vi "Handle Last Ack Core.vi"(4 "error in (no error)":errorcluster, 6 "Last Ack":refnum<class "Last Ack.lvclass">, 7 "Controller in":refnum<class "Controller.lvclass">) -> (0 "error out":errorcluster, 3 "Controller out":refnum<class "Controller.lvclass">)   [LabVIEW 2016, in "Controller Actor.lvlib" / "Controller.lvclass"]
doc: "(<B>Filename</B>: Actor Framework.lvlib:Actor.lvclass:Handle Last Ack Core.vi)\n\nDefines how the caller actor responds to the Last Ack message from a nested actor. The Last Ack message is the final message a nested actor sends to its caller before it shuts down. The message contains information about the final state of the nested actor.\n\nBy default, this method does nothing except return any error the nested actor sent. A descendant class may override this method to define behavior."
uses:
  Controller.lvclass
  <vilib>/ActorFramework/LastAck/Last Ack.lvclass
  <vilib>/ActorFramework/LastAck/Last Ack.lvclass/Last Ack.ctl
  Hardware/HW Config/HW Configuration.lvclass
  Hardware/Hardware.lvclass
  Hardware/HW Config/HW Configuration.lvclass/HW Configuration.ctl
  Hardware/Hardware.lvclass/Hardware.ctl
  Controller.lvclass/Controller.ctl
  <userlib>/Configuration Dialog Actor/Configuration.lvclass
  <vilib>/ActorFramework/Message Enqueuer/Message Enqueuer.lvclass/Message Enqueuer.ctl
  Measurement Actor/Measurement.lvclass
  Measurement Actor/Measurement.lvclass/Measurement.ctl
  <vilib>/ActorFramework/Message Enqueuer/Enqueue.vi
  User Interface/Messages/Enable UI Msg/Enable UI Msg.lvclass
  C:/Program Files (x86)/National Instruments/LabVIEW 2016/vi.lib/ActorFramework/Message/Message.lvclass
  <vilib>/ActorFramework/Message Priority Queue/Priority Enqueue.vi
  <vilib>/ActorFramework/Actor/Actor.lvclass
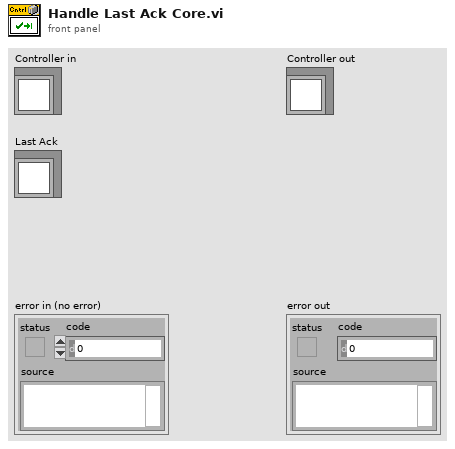
[diagram p1: front panel]
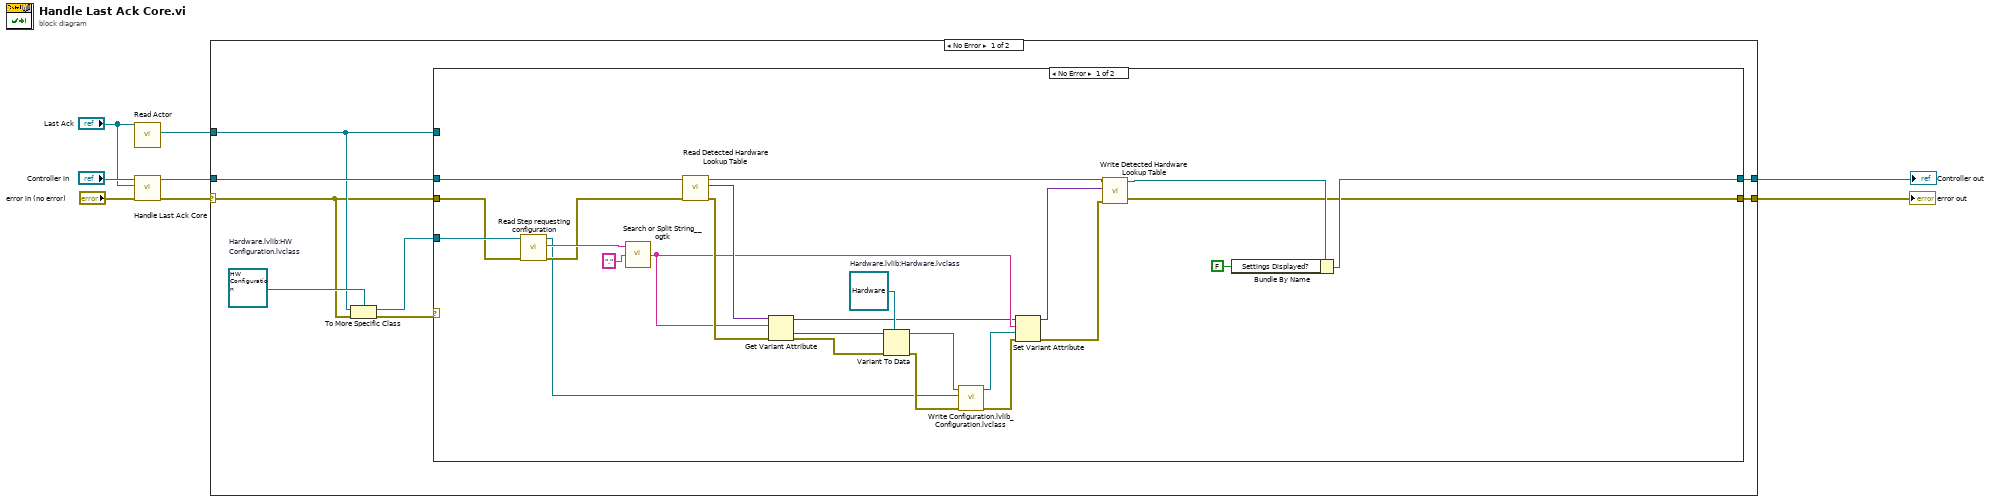
[diagram p0: block diagram]
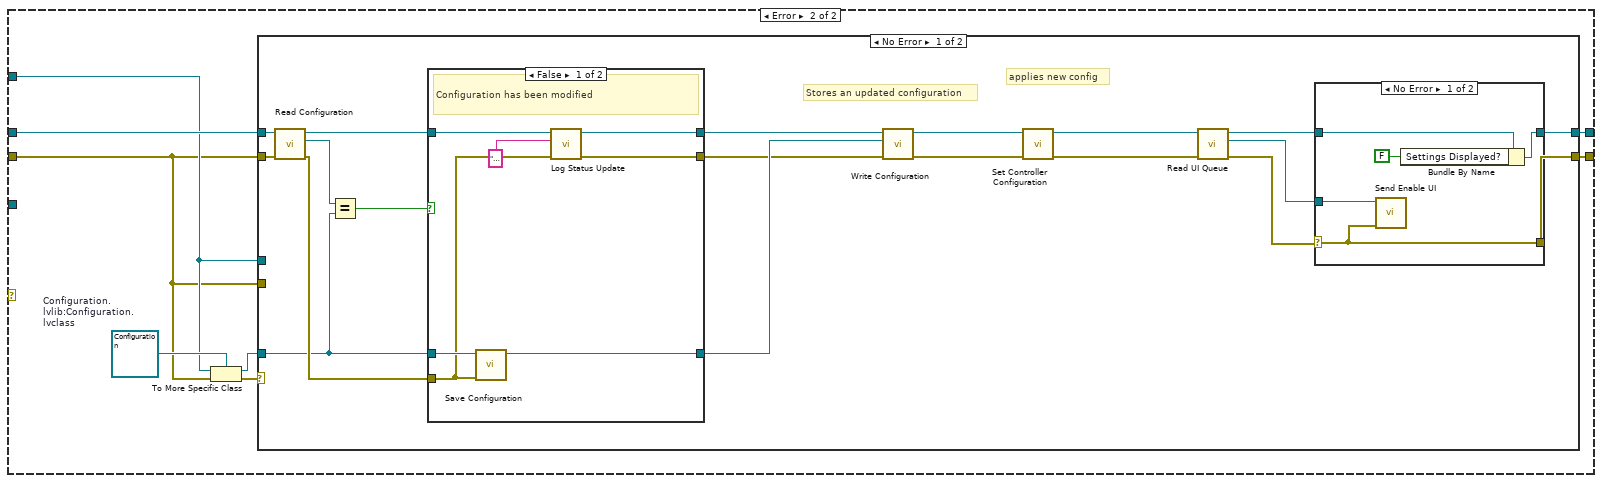
[diagram p2: hidden frame]
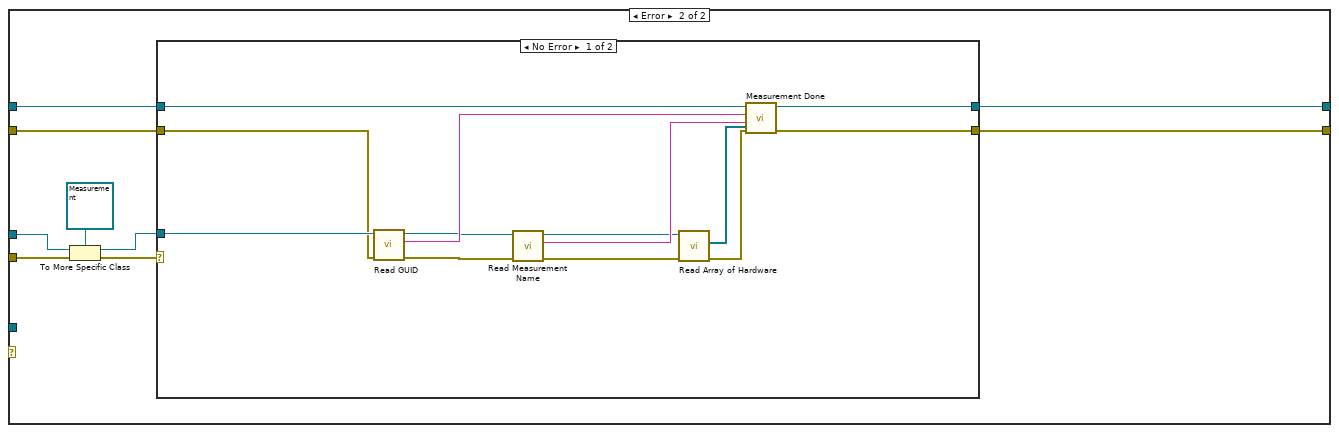
[diagram p5: hidden frame]
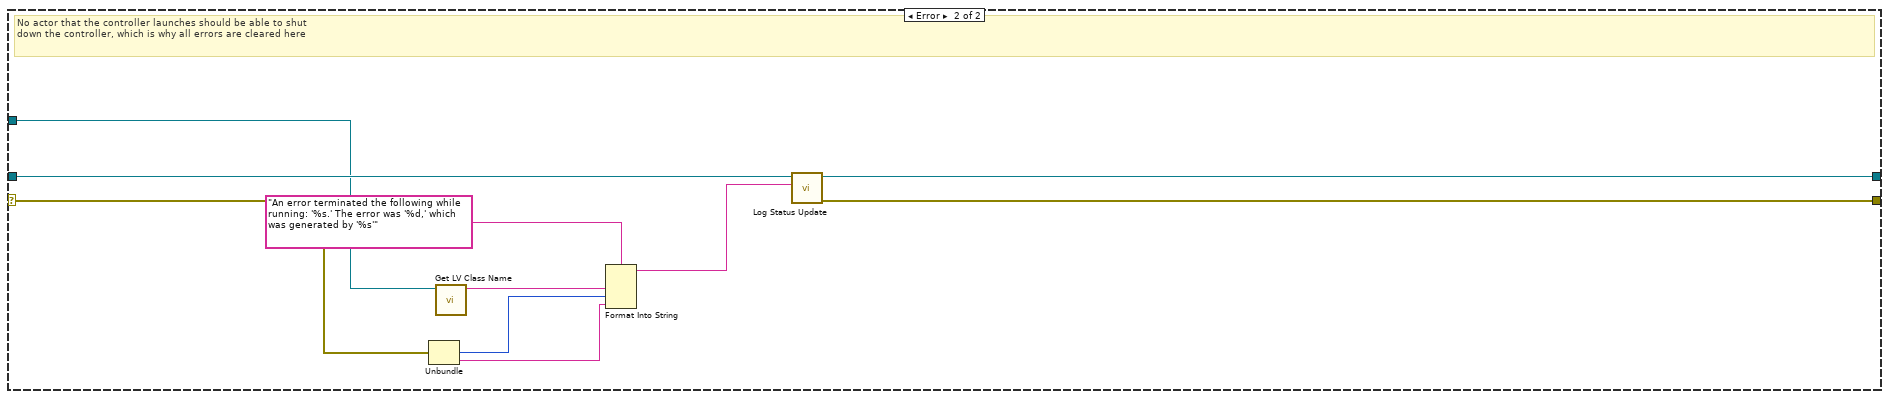
[diagram p7: hidden frame]
diagram:
  n1 = call <vilib>:"Read Actor.vi"("Last Ack"="Last Ack") -> ("Actor"=w3:refnum<class "Actor.lvclass">)  [unwired: 10 in]
  n2 = call-parent "Handle Last Ack Core.vi"("error in (no error)"="error in (no error)", "Last Ack"="Last Ack", "Actor in"="Controller in") -> ("error out"=w2:errorcluster, "Actor out"=w4:refnum<class "Controller.lvclass">)  [unwired: 3 in]
  n3 = case shown="No Error" w2 {
    selector: w2 -> [w9 w115]
    tunnel: [w16 w118] -> w7
    tunnel: [w15 w117] -> w5
    tunnel: w4 -> [w14 w119]
    tunnel: w3 -> [w12 w111]
    frame No Error {
      w13 = refnum<class "HW Configuration.lvclass"> refnum  # Hardware.lvlib:HW Configuration.lvclass
      n4 = To More Specific Class(target class=w13, reference=w12, error in=w9) -> (specific class reference=w11:refnum<class "HW Configuration.lvclass">, error out=w10:errorcluster)
      n5 = case shown="No Error" w10 {
        tunnel: [w19 w49] -> w16
        tunnel: [w18 w48] -> w15
        tunnel: w14 -> [w34 w47]
        tunnel: w12 -> [_ w43]
        tunnel: w9 -> [w40 w42]
        tunnel: w11 -> [w41 _]
        frame No Error {
          w32 = refnum<class "Hardware.lvclass"> refnum  # Hardware.lvlib:Hardware.lvclass
          n6 = call "Read Step requesting configuration.vi"("error in (no error)"=w40, "HW Configuration in"=w41) -> ("error out"=w35:errorcluster, "Step requesting configuration"=w39:string, "HW Configuration out"=w17:refnum<class "HW Configuration.lvclass">)  [unwired: 7 in]
          n7 = call <userlib>:"Search or Split String__ogtk.vi"("search string/char (-)"="." ("regular expression"), "string"=w39) -> ("substring after match"=w28:string)  [unwired: 1 in, 2 out]
          n8 = call "Read Detected Hardware Lookup Table.vi"("error in (no error)"=w35, "Controller in"=w34) -> ("error out"=w36:errorcluster, "Detected Hardware Lookup Table"=w37:variant, "Controller out"=w23:refnum<class "Controller.lvclass">)  [unwired: 7 in]
          n9 = Get Variant Attribute(Variant=w37, name=w28, error in=w36) -> (duplicate Variant=w27:variant, value=w33:variant, error out=w31:errorcluster)  [unwired: 1 in, 1 out]
          n10 = Variant To Data(error in=w31, type=w32, Variant=w33) -> (data=w30:refnum<class "Hardware.lvclass">, error out=w25:errorcluster)
          n11 = call "Write Configuration.lvlib_Configuration.lvclass.vi"("error in (no error)"=w25, "Hardware.lvlib:HW Configuration.lvclass"=w17, "Hardware in"=w30) -> ("error out"=w26:errorcluster, "Hardware out"=w29:refnum<class "Hardware.lvclass">)  [unwired: 7 in]
          n12 = Set Variant Attribute(Variant=w27, name=w28, value=w29, error in=w26) -> (Variant out=w24:variant, error out=w20:errorcluster)  [unwired: 1 out]
          n13 = call "Write Detected Hardware Lookup Table.vi"("error in (no error)"=w20, "Detected Hardware Lookup Table"=w24, "Controller in"=w23) -> ("error out"=w18:errorcluster, "Controller out"=w22:refnum<class "Controller.lvclass">)  [unwired: 7 in]
          n14 = Bundle By Name(cluster=w22, "Settings Displayed?"=FALSE) -> (w19:refnum<class "Controller.lvclass">)
        }
        frame Error {
          w44 = refnum<class "Configuration.lvclass"> refnum  # Configuration.lvlib:Configuration.lvclass
          n15 = To More Specific Class(target class=w44, reference=w43, error in=w42) -> (specific class reference=w46:refnum<class "Configuration.lvclass">, error out=w45:errorcluster)
          n16 = case shown="No Error" w45 {
            tunnel: [w63 w87] -> w49
            tunnel: [w60 w86] -> w48
            tunnel: w47 -> [w58 w89]
            tunnel: w46 -> [w55 _]
            tunnel: w42 -> [w53 w88]
            tunnel: w43 -> [_ w94]
            tunnel: w42 -> [_ w93]
            frame No Error {
              # "applies new config"
              # "Stores an updated configuration"
              n17 = call "Read Configuration.vi"("error in (no error)"=w53, "Controller in"=w58) -> ("error out"=w57:errorcluster, "Configuration.lvlib:Configuration.lvclass"=w56:refnum<class "Configuration.lvclass">, "Controller out"=w52:refnum<class "Controller.lvclass">)  [unwired: 7 in]
              n18 = Equal?(x=w56, y=w55) -> (x = y?=w54:bool)
              n19 = case shown="False" w54 {
                tunnel: w55 -> [w75 w78]
                tunnel: [w74 w78] -> w59
                tunnel: w57 -> [w70 w76]
                tunnel: w52 -> [w73 w77]
                tunnel: [w72 w77] -> w51
                tunnel: [w69 w76] -> w50
                frame False {
                  # "Configuration has been modified"
                  n20 = call <userlib>:"Save Configuration.vi"("error in (no error)"=w70, "Configuration in"=w75) -> ("Configuration out"=w74:refnum<class "Configuration.lvclass">)  [unwired: 7 in, 2 out]
                  n21 = call-dynamic "Log Status Update.vi"("error in (no error)"=w70, "String"="Settings updated and saved to disk without error", "Controller in"=w73) -> ("error out"=w69:errorcluster, "Controller out"=w72:refnum<class "Controller.lvclass">)  [unwired: 7 in]
                }
                frame True {
                }
              }
              n22 = call "Write Configuration.vi"("error in (no error)"=w50, "Configuration.lvlib:Configuration.lvclass"=w59, "Controller in"=w51) -> ("error out"=w68:errorcluster, "Controller out"=w67:refnum<class "Controller.lvclass">)  [unwired: 7 in]
              n23 = call-dynamic "Set Controller Configuration.vi"("error in (no error)"=w68, "Controller in"=w67) -> ("error out"=w62:errorcluster, "Controller out"=w66:refnum<class "Controller.lvclass">)  [unwired: 8 in]
              n24 = call "Read UI Queue.vi"("error in (no error)"=w62, "UI Controller in"=w66) -> ("error out"=w61:errorcluster, "UI Queue"=w65:refnum<class "Message Enqueuer.lvclass">, "UI Controller out"=w64:refnum<class "Controller.lvclass">)  [unwired: 7 in]
              n25 = case shown="No Error" w61 {
                selector: w61 -> [w79 w84]
                tunnel: w65 -> [w83 _]
                tunnel: w64 -> [w82 w85]
                tunnel: [w80 w85] -> w63
                tunnel: [w79 w84] -> w60
                frame No Error {
                  n26 = call "Send Enable UI.vi"("error in (no error)"=w79, "Message Enqueuer"=w83) -> ()  [unwired: 8 in, 2 out]
                  n27 = Bundle By Name(cluster=w82, "Settings Displayed?"=FALSE) -> (w80:refnum<class "Controller.lvclass">)
                }
                frame Error {
                }
              }
            }
            frame Error {
              n28 = To More Specific Class(target class=refnum<class "Measurement.lvclass"> refnum ("Measurement Actor.lvlib:Measurement.lvclass"), reference=w94, error in=w93) -> (specific class reference=w90:refnum<class "Measurement.lvclass">, error out=w91:errorcluster)
              n29 = case shown="No Error" w91 {
                tunnel: w90 -> [w101 _]
                tunnel: w89 -> [w107 w109]
                tunnel: w88 -> [w97 w108]
                tunnel: [w106 w109] -> w87
                tunnel: [w105 w108] -> w86
                frame No Error {
                  n30 = call "Read GUID.vi"("error in (no error)"=w97, "Measurement in"=w101) -> ("error out"=w96:errorcluster, "GUID"=w103:string, "Measurement out"=w100:refnum<class "Measurement.lvclass">)  [unwired: 7 in]
                  n31 = call "Read Measurement Name.vi"("error in (no error)"=w96, "Measurement in"=w100) -> ("error out"=w95:errorcluster, "Measurement Name"=w102:string, "Measurement out"=w99:refnum<class "Measurement.lvclass">)  [unwired: 7 in]
                  n32 = call "Read Array of Hardware.vi"("error in (no error)"=w95, "Measurement in"=w99) -> ("error out"=w98:errorcluster, "Array of Hardware"=w104:refnum<class "Hardware.lvclass">[])  [unwired: 7 in, 1 out]
                  n33 = call-dynamic "Measurement Done.vi"("Array of Hardware"=w104, "error in (no error)"=w98, "Measurement Name"=w102, "GUID"=w103, "Controller in"=w107) -> ("error out"=w105:errorcluster, "Controller out"=w106:refnum<class "Controller.lvclass">)  [unwired: 5 in]
                }
                frame Error {
                }
              }
            }
          }
        }
      }
    }
    frame Error {
      # "No actor that the controller launches should be able to shut\ndown the controller, which is why all errors are cleared here"
      n34 = Unbundle(w115) -> ("code"=w113:i32, "source"=w112:string)  [unwired: 1 out]
      n35 = call <vilib>:"Get LV Class Name.vi"("object"=w111) -> ("class name"=w110:string)  [unwired: 9 in, 1 out]
      n36 = Format Into String(format string="An error terminated the following while running: '%s.' The error was '%d,' which was generated by '%s'", w110, w113, w112) -> (resulting string=w116:string)  [unwired: 2 in, 1 out]
      n37 = call-dynamic "Log Status Update.vi"("String"=w116, "Controller in"=w119) -> ("error out"=w117:errorcluster, "Controller out"=w118:refnum<class "Controller.lvclass">)  [unwired: 8 in]
    }
  }
  "Controller out" <- w7
  "error out" <- w5
